vi "Create Server from Template.vi"(8 "error in (no error)":errorcluster, 9 "Generated Server Name":string="Generated Server", 10 "Target Project Path":path, 11 "Application ref in":refnum<vi>) -> (0 "error out":errorcluster, 1 "Already exists ?":bool, 2 "Server class out":refnum<vi>, 3 "Server library out":refnum<vi>)   [LabVIEW 2019, in "gRPC Scripting Tools.lvlib"]
uses:
  gRPC Scripting Tools.lvlib
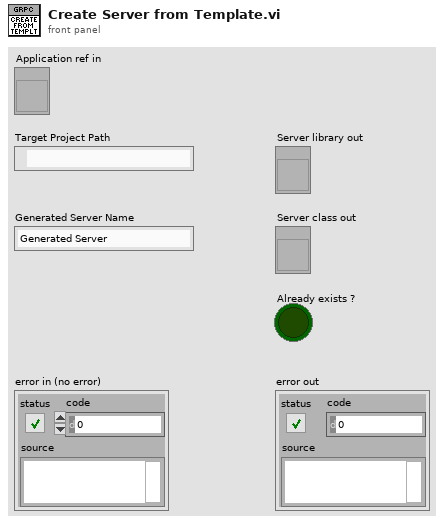
[diagram p1: front panel]
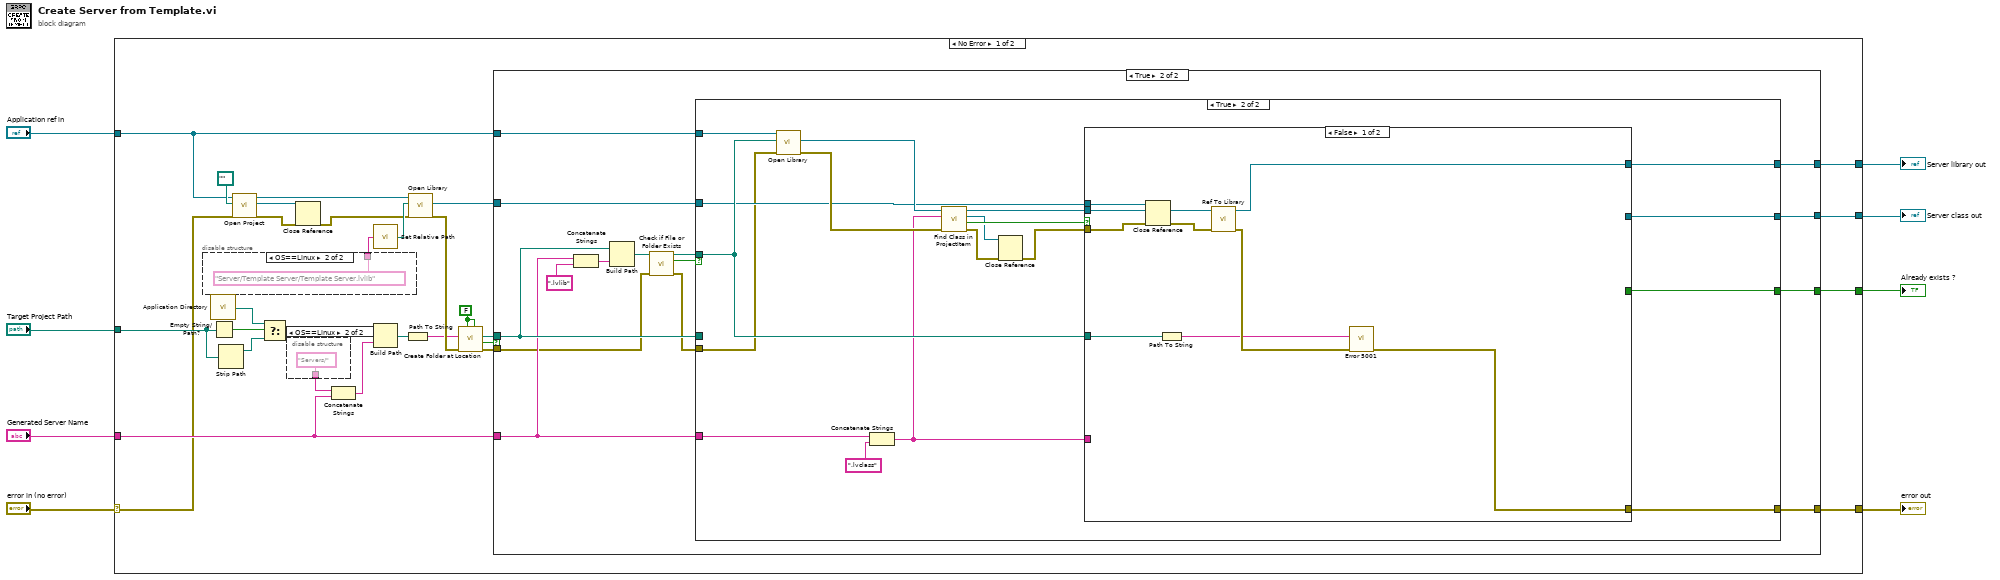
[diagram p0: block diagram]
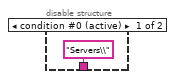
[diagram p2: hidden frame]
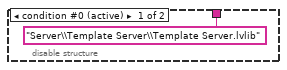
[diagram p3: hidden frame]
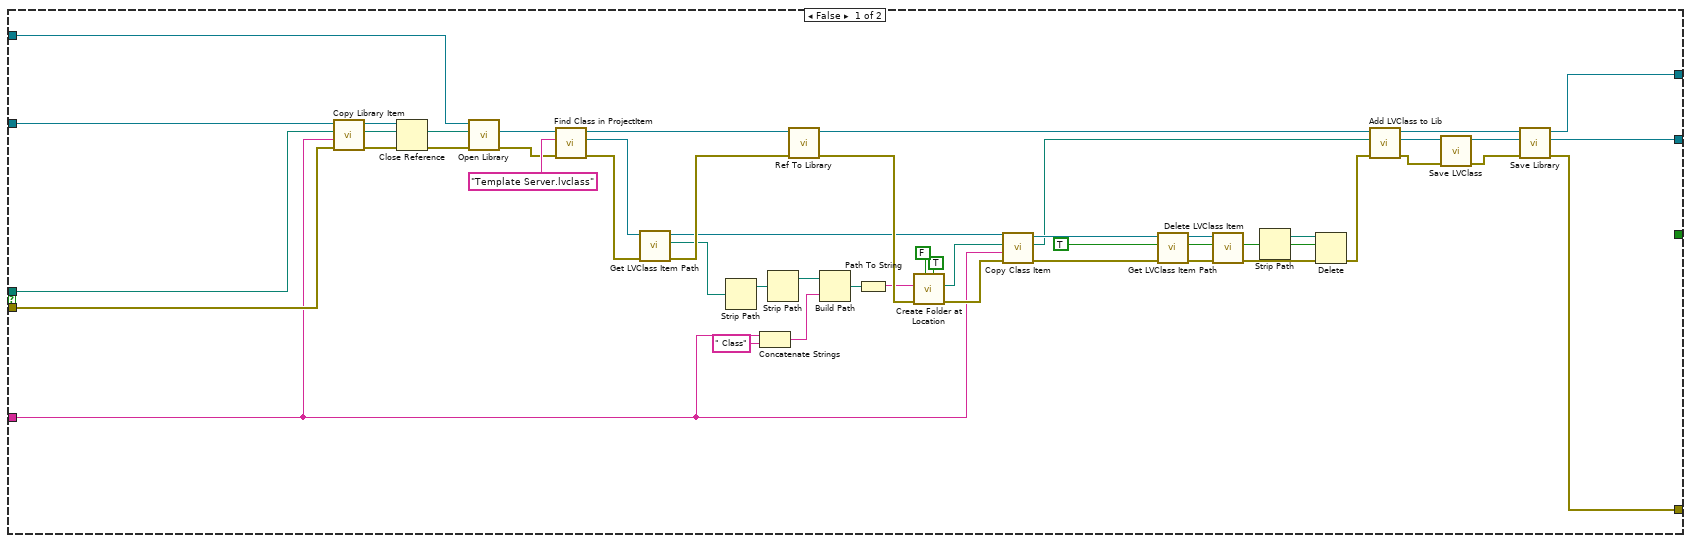
[diagram p4: hidden frame]
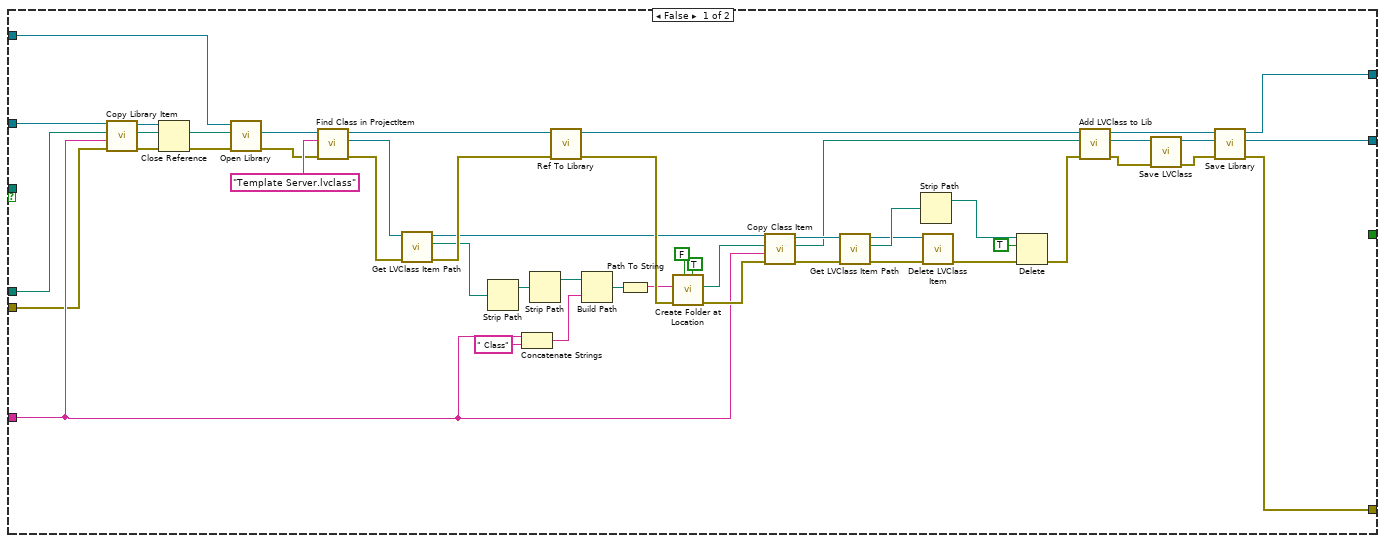
[diagram p5: hidden frame]
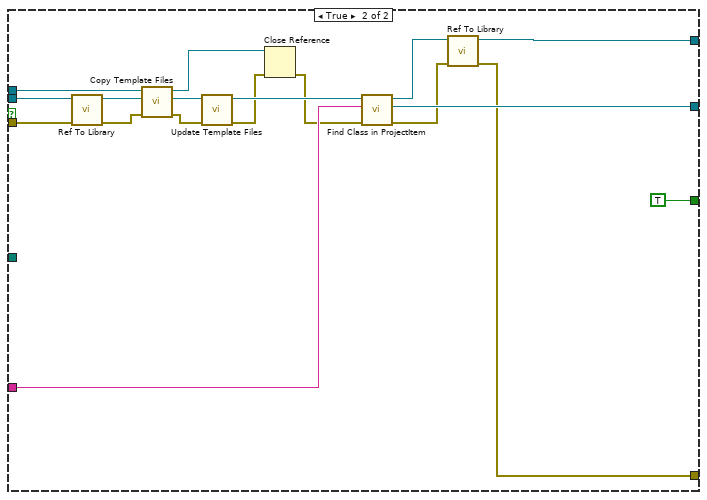
[diagram p6: hidden frame]
diagram:
  n1 = case shown="No Error" "error in (no error)" {
    selector: "error in (no error)" -> [w11 w196]
    tunnel: [w37 w196] -> w8
    tunnel: [w36 _] -> w7
    tunnel: [w35 _] -> w6
    tunnel: "Target Project Path" -> [w14 _]
    tunnel: "Generated Server Name" -> [w13 _]
    tunnel: "Application ref in" -> [w12 _]
    tunnel: [w9 _] -> w1
    frame No Error {
      w27 = FALSE ("Use Relative")
      n2 = disable-structure shown="OS==Linux" {
        disable-tunnel: ["Server\\Template Server\\Template Server.lvlib" ("Application Relative Path") "Server/Template Server/Template Server.lvlib" ("Application Relative Path")] -> w28
        frame condition #0 (active) {
        }
        frame condition #1 {
        }
      }
      n3 = call <vilib>:"Application Directory.vi"() -> ("Application Directory"=w15:path)
      n4 = Empty String/Path?(string/path=w14) -> (empty?=w18:bool)
      n5 = Strip Path(path=w14) -> (stripped path=w17:path)  [unwired: 1 out]
      n6 = call "Open Project.vi"("error in (no error)"=w11, "Project Path in"=path "", "Application reference"=w12) -> ("error out"=w21:errorcluster, "Project out"=w22:refnum<vi>, "Application out"=w31:refnum<vi>)  [unwired: 6 in]
      n7 = Select(t=w15, s=w18, f=w17) -> (s? t:f=w16:path)
      n8 = disable-structure shown="OS==Linux" {
        disable-tunnel: ["Servers\\" ("Path") "Servers/" ("Path")] -> w26
        frame condition #0 (active) {
        }
        frame condition #1 {
        }
      }
      n9 = Close Reference(reference=w22, error in (no error)=w21) -> (error out=w20:errorcluster)
      n10 = Concatenate Strings(w26, w13) -> (w25:string)
      n11 = call "Set Relative Path.vi"("Application Relative Path"=w28) -> ("Full Path"=w32:path)
      n12 = Build Path(base path=w16, name or relative path=w25) -> (appended path=w24:path)
      n13 = Path To String(path=w24) -> (string=w23:string)
      n14 = call "Open Library.vi"("error in (no error)"=w20, "Full Path"=w32, "Application in"=w31) -> ("error out"=w33:errorcluster, "Library out"=w29:refnum<vi>)  [unwired: 6 in, 1 out]
      n15 = call "Create Folder at Location.vi"("Override existing (F)"=w27, "Use Relative (F)"=w27, "Error In"=w33, "Path"=w23) -> ("Error Out"=w34:errorcluster, "Already Exists ?"=w10:bool, "Full path out"=w30:path)  [unwired: 5 in]
      n16 = case shown="True" w10 {
        tunnel: [w88 w93] -> w37
        tunnel: [w87 w98] -> w36
        tunnel: [w86 w99] -> w35
        tunnel: w34 -> [w50 w90]
        tunnel: w30 -> [w49 w95]
        tunnel: w29 -> [w48 w96]
        tunnel: w13 -> [w43 w94]
        tunnel: w12 -> [w42 w97]
        tunnel: [_ w92] -> w9
        frame False {
          n17 = call "Copy Library Item.vi"("error in (no error)"=w50, "Copy Name"=w43, "Copy location"=w49, "Library in"=w48) -> ("error out"=w71:errorcluster, "New Lib Path"=w47:path, "Library out"=w70:refnum<vi>)  [unwired: 5 in]
          n18 = Close Reference(reference=w70, error in (no error)=w71) -> (error out=w46:errorcluster)
          n19 = call "Open Library.vi"("error in (no error)"=w46, "Full Path"=w47, "Application in"=w42) -> ("error out"=w44:errorcluster, "Library out"=w45:refnum<vi>)  [unwired: 6 in, 1 out]
          n20 = call "Find Class in ProjectItem.vi"("error in (no error)"=w44, "Class Name"="Template Server.lvclass", "ProjectItem in"=w45) -> ("error out"=w53:errorcluster, "LVClass out"=w52:refnum<vi>, "ProjectItem out"=w65:refnum<vi>)  [unwired: 5 in, 1 out]
          n21 = call "Get LVClass Item Path.vi"("error in (no error)"=w53, "LVClassLibrary in"=w52) -> ("error out"=w67:errorcluster, "Path"=w54:path, "LVClassLibrary out"=w55:refnum<vi>)  [unwired: 7 in]
          n22 = Strip Path(path=w54) -> (stripped path=w63:path)  [unwired: 1 out]
          n23 = Concatenate Strings(w43, " Class" ("string")) -> (w58:string)
          n24 = Strip Path(path=w63) -> (stripped path=w64:path)  [unwired: 1 out]
          n25 = call "Ref To Library.vi"("error in (no error)"=w67, "ProjectItem in"=w65) -> ("error out"=w68:errorcluster, "Library out"=w81:refnum<vi>)  [unwired: 8 in]
          n26 = Build Path(base path=w64, name or relative path=w58) -> (appended path=w59:path)
          n27 = Path To String(path=w59) -> (string=w60:string)
          n28 = call "Create Folder at Location.vi"("Override existing (F)"=TRUE, "Use Relative (F)"=FALSE ("Use Relative"), "Error In"=w68, "Path"=w60) -> ("Error Out"=w69:errorcluster, "Full path out"=w62:path)  [unwired: 5 in, 1 out]
          n29 = call "Copy Class Item.vi"("error in (no error)"=w69, "New Name"=w43, "Full path in"=w62, "LVClassLibrary in"=w55) -> ("error out"=w73:errorcluster, "New Class Path out"=w66:path, "LVClassLibrary out"=w72:refnum<vi>)  [unwired: 5 in]
          n30 = call "Get LVClass Item Path.vi"("error in (no error)"=w73, "LVClassLibrary in"=w72) -> ("error out"=w75:errorcluster, "Path"=w76:path, "LVClassLibrary out"=w74:refnum<vi>)  [unwired: 7 in]
          n31 = call "Delete LVClass Item.vi"("error in (no error)"=w75, "LVClassLibrary in"=w74) -> ("error out"=w78:errorcluster)  [unwired: 9 in]
          n32 = Strip Path(path=w76) -> (stripped path=w77:path)  [unwired: 1 out]
          n33 = Delete(path (use dialog)=w77, entire hierarchy (F)=TRUE, error in=w78) -> (error out=w79:errorcluster)  [unwired: 2 in, 2 out]
          n34 = call "Add LVClass to Lib.vi"("error in (no error)"=w79, "LVClass Path in"=w66, "Library in"=w81) -> ("error out"=w84:errorcluster, "LVClassLibrary out"=w83:refnum<vi>, "Library out"=w82:refnum<vi>)  [unwired: 6 in]
          n35 = call "Save LVClass.vi"("error in (no error)"=w84, "LVClassLibrary in"=w83) -> ("error out"=w85:errorcluster, "LVClassLibrary out"=w87:refnum<vi>)  [unwired: 8 in]
          n36 = call "Save Library.vi"("error in (no error)"=w85, "Library in"=w82) -> ("error out"=w88:errorcluster, "Library out"=w86:refnum<vi>)  [unwired: 8 in]
        }
        frame True {
          n37 = Concatenate Strings(w94, ".lvlib" ("string")) -> (w102:string)
          n38 = Build Path(base path=w95, name or relative path=w102) -> (appended path=w101:path)
          n39 = call <vilib>:"Check if File or Folder Exists.vi"("error in (no error)"=w90, "path"=w101) -> ("error out"=w89:errorcluster, "file or folder exists?"=w100:bool, "dup path"=w91:path)  [unwired: 7 in]
          n40 = case shown="True" w100 {
            tunnel: [w111 w162] -> w99
            tunnel: [w110 w151] -> w98
            tunnel: w97 -> [w109 w168]
            tunnel: w96 -> [w108 w157]
            tunnel: w95 -> [w107 _]
            tunnel: w94 -> [w106 w166]
            tunnel: w89 -> [w105 w156]
            tunnel: [w104 w161] -> w93
            tunnel: [_ w159] -> w92
            tunnel: w91 -> [_ w158]
            frame False {
              n41 = call "Copy Library Item.vi"("error in (no error)"=w105, "Copy Name"=w106, "Copy location"=w107, "Library in"=w108) -> ("error out"=w136:errorcluster, "New Lib Path"=w115:path, "Library out"=w135:refnum<vi>)  [unwired: 5 in]
              n42 = Close Reference(reference=w135, error in (no error)=w136) -> (error out=w114:errorcluster)
              n43 = call "Open Library.vi"("error in (no error)"=w114, "Full Path"=w115, "Application in"=w109) -> ("error out"=w112:errorcluster, "Library out"=w113:refnum<vi>)  [unwired: 6 in, 1 out]
              n44 = call "Find Class in ProjectItem.vi"("error in (no error)"=w112, "Class Name"="Template Server.lvclass", "ProjectItem in"=w113) -> ("error out"=w118:errorcluster, "LVClass out"=w117:refnum<vi>, "ProjectItem out"=w130:refnum<vi>)  [unwired: 5 in, 1 out]
              n45 = call "Get LVClass Item Path.vi"("error in (no error)"=w118, "LVClassLibrary in"=w117) -> ("error out"=w132:errorcluster, "Path"=w119:path, "LVClassLibrary out"=w120:refnum<vi>)  [unwired: 7 in]
              n46 = Strip Path(path=w119) -> (stripped path=w128:path)  [unwired: 1 out]
              n47 = Concatenate Strings(w106, " Class" ("string")) -> (w123:string)
              n48 = Strip Path(path=w128) -> (stripped path=w129:path)  [unwired: 1 out]
              n49 = call "Ref To Library.vi"("error in (no error)"=w132, "ProjectItem in"=w130) -> ("error out"=w133:errorcluster, "Library out"=w146:refnum<vi>)  [unwired: 8 in]
              n50 = Build Path(base path=w129, name or relative path=w123) -> (appended path=w124:path)
              n51 = Path To String(path=w124) -> (string=w125:string)
              n52 = call "Create Folder at Location.vi"("Override existing (F)"=TRUE, "Use Relative (F)"=FALSE ("Use Relative"), "Error In"=w133, "Path"=w125) -> ("Error Out"=w134:errorcluster, "Full path out"=w127:path)  [unwired: 5 in, 1 out]
              n53 = call "Copy Class Item.vi"("error in (no error)"=w134, "New Name"=w106, "Full path in"=w127, "LVClassLibrary in"=w120) -> ("error out"=w138:errorcluster, "New Class Path out"=w131:path, "LVClassLibrary out"=w137:refnum<vi>)  [unwired: 5 in]
              n54 = call "Get LVClass Item Path.vi"("error in (no error)"=w138, "LVClassLibrary in"=w137) -> ("error out"=w140:errorcluster, "Path"=w141:path, "LVClassLibrary out"=w139:refnum<vi>)  [unwired: 7 in]
              n55 = Strip Path(path=w141) -> (stripped path=w142:path)  [unwired: 1 out]
              n56 = call "Delete LVClass Item.vi"("error in (no error)"=w140, "LVClassLibrary in"=w139) -> ("error out"=w143:errorcluster)  [unwired: 9 in]
              n57 = Delete(path (use dialog)=w142, entire hierarchy (F)=TRUE, error in=w143) -> (error out=w144:errorcluster)  [unwired: 2 in, 2 out]
              n58 = call "Add LVClass to Lib.vi"("error in (no error)"=w144, "LVClass Path in"=w131, "Library in"=w146) -> ("error out"=w149:errorcluster, "LVClassLibrary out"=w148:refnum<vi>, "Library out"=w147:refnum<vi>)  [unwired: 6 in]
              n59 = call "Save LVClass.vi"("error in (no error)"=w149, "LVClassLibrary in"=w148) -> ("error out"=w150:errorcluster, "LVClassLibrary out"=w110:refnum<vi>)  [unwired: 8 in]
              n60 = call "Save Library.vi"("error in (no error)"=w150, "Library in"=w147) -> ("error out"=w104:errorcluster, "Library out"=w111:refnum<vi>)  [unwired: 8 in]
            }
            frame True {
              n61 = call "Open Library.vi"("error in (no error)"=w156, "Full Path"=w158, "Application in"=w168) -> ("error out"=w164:errorcluster, "Library out"=w167:refnum<vi>)  [unwired: 6 in, 1 out]
              n62 = Concatenate Strings(w166, ".lvclass" ("Class Name")) -> (w152:string)
              n63 = call "Find Class in ProjectItem.vi"("error in (no error)"=w164, "Class Name"=w152, "ProjectItem in"=w167) -> ("error out"=w154:errorcluster, "Found?"=w160:bool, "LVClass out"=w155:refnum<vi>, "ProjectItem out"=w163:refnum<vi>)  [unwired: 5 in]
              n64 = Close Reference(reference=w155, error in (no error)=w154) -> (error out=w153:errorcluster)
              n65 = case shown="False" w160 {
                tunnel: w163 -> [w177 w190]
                tunnel: [w176 w195] -> w162
                tunnel: w153 -> [w171 w192]
                tunnel: [w174 w183] -> w161
                tunnel: w158 -> [w173 _]
                tunnel: [_ TRUE] -> w159
                tunnel: w157 -> [w172 w182]
                tunnel: w152 -> [_ w189]
                tunnel: [_ w188] -> w151
                frame False {
                  n66 = Close Reference(reference=w172, error in (no error)=w171) -> (error out=w170:errorcluster)
                  n67 = Path To String(path=w173) -> (string=w169:string)
                  n68 = call "Ref To Library.vi"("error in (no error)"=w170, "ProjectItem in"=w177) -> ("error out"=w175:errorcluster, "Library out"=w176:refnum<vi>)  [unwired: 8 in]
                  n69 = call "Error 5001.vi"("error in (no error)"=w175, "Server Class Path"=w169) -> ("error out"=w174:errorcluster)  [unwired: 9 in]
                }
                frame True {
                  n70 = call "Ref To Library.vi"("error in (no error)"=w192, "ProjectItem in"=w190) -> ("error out"=w191:errorcluster, "Library out"=w193:refnum<vi>)  [unwired: 8 in]
                  n71 = call "Copy Template Files.vi"("error in (no error)"=w191, "Server Library (Library Item) in"=w193, "Template Library (Library Item) in"=w182) -> ("error out"=w181:errorcluster, "Server Library (Library Item) out"=w180:refnum<vi>, "Template Library (Library Item) out"=w178:refnum<vi>)  [unwired: 6 in]
                  n72 = call "Update Template Files.vi"("error in (no error)"=w181, "Server Library (Library Item) in"=w180) -> ("error out"=w179:errorcluster, "Server Library (Library Item) out"=w187:refnum<vi>)  [unwired: 8 in]
                  n73 = Close Reference(reference=w178, error in (no error)=w179) -> (error out=w185:errorcluster)
                  n74 = call "Find Class in ProjectItem.vi"("error in (no error)"=w185, "Class Name"=w189, "ProjectItem in"=w187) -> ("error out"=w184:errorcluster, "LVClass out"=w188:refnum<vi>, "ProjectItem out"=w186:refnum<vi>)  [unwired: 5 in, 1 out]
                  n75 = call "Ref To Library.vi"("error in (no error)"=w184, "ProjectItem in"=w186) -> ("error out"=w183:errorcluster, "Library out"=w195:refnum<vi>)  [unwired: 8 in]
                }
              }
            }
          }
        }
      }
    }
    frame Error {
    }
  }
  "error out" <- w8
  "Server class out" <- w7
  "Server library out" <- w6
  "Already exists ?" <- w1
